vi "FPGA_target_execute_function.vi"(0 "tick_count_in":u32, 2 "data_in":T1, 4 "set_stop_output_in":bool, 5 "input_data_in":u8, 7 "stop_request":bool, 8 "fifo_empty_in":bool, 11 "C1_data":T2) -> (10 "set_output":bool, 12 "read_fifo":bool, 13 "stop":bool, 14 "tick_count_out":u32, 16 "data_dup":T1, 17 "fifo_empty_out":bool, 18 "set_stop_output_out":bool, 19 "input_data_out":u8)   [LabVIEW 2014]
doc: "executes a command (time, wait, jump, stop)"
uses:
  FPGA_32BitPattern_data_type.ctl
  FPGA_cmd_data_type.ctl
  <vilib>/rvi/eio/common/nirviEmuTemplateMethod_errors.vi
  <vilib>/eio/EIONode/EIONode.xnode
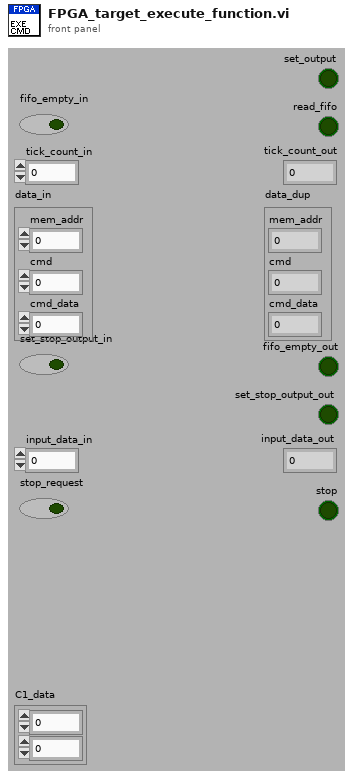
[diagram p1: front panel]
types:
  T1 = typedef "FPGA_cmd_data_type.ctl" = cluster{"mem_addr":u32, "cmd":u8, "cmd_data":u32}
  T2 = typedef "FPGA_32BitPattern_data_type.ctl" = cluster{"port0":u8, "port1":u8}
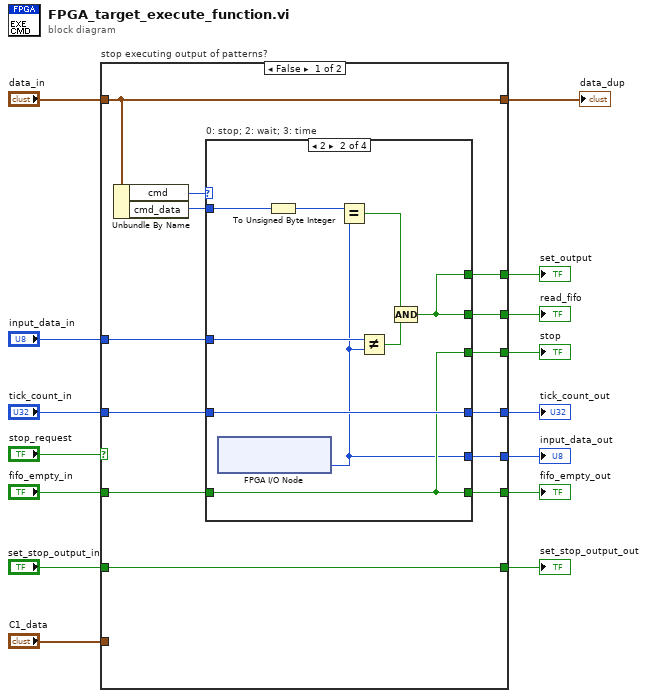
[diagram p0: block diagram]
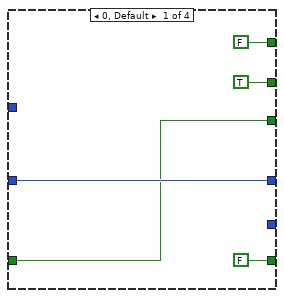
[diagram p2: hidden frame]
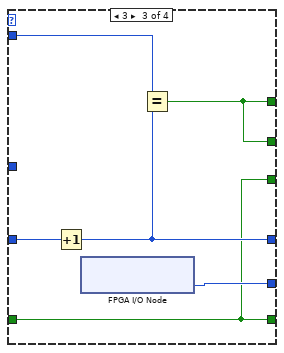
[diagram p3: hidden frame]
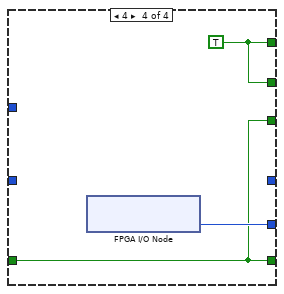
[diagram p4: hidden frame]
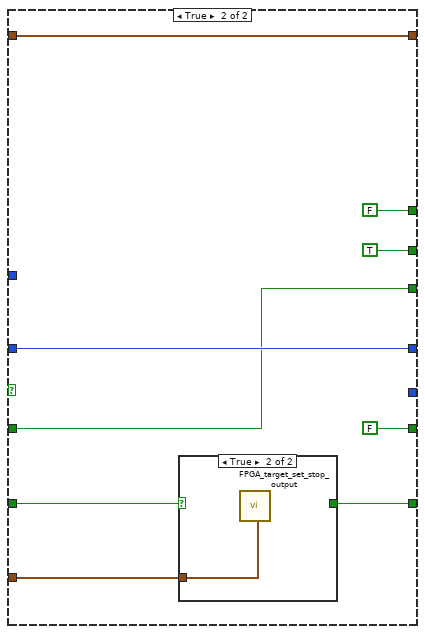
[diagram p5: hidden frame]
diagram:
  n1 = case "stop executing output of patterns?" shown="False" "stop_request" {
    tunnel: "tick_count_in" -> [w28 w59]
    tunnel: [w27 FALSE] -> w14
    tunnel: [w26 w59] -> w13
    tunnel: [w25 w53] -> w12
    tunnel: "fifo_empty_in" -> [w21 w53]
    tunnel: [w16 TRUE] -> w9
    tunnel: [w24 _] -> w8
    tunnel: "input_data_in" -> [w23 _]
    tunnel: "set_stop_output_in" -> [w22 w57]
    tunnel: "C1_data" -> [_ w56]
    tunnel: [w22 w55] -> w4
    tunnel: "data_in" -> [w20 w54]
    tunnel: [w20 w54] -> w2
    tunnel: [w17 FALSE ("fifo_empty_in")] -> w1
    frame False {
      n2 = Unbundle By Name(w20) -> ("cmd"=w19:u8, "cmd_data"=w18:u32)
      n3 = case "0: stop; 2: wait; 3: time" shown="2" w19 {
        tunnel: w18 -> [_ w39 w48 _]
        tunnel: w28 -> [w33 w42 w46 _]
        tunnel: [FALSE w36 w43 w49] -> w27
        tunnel: [w33 w42 w45 _] -> w26
        tunnel: [w31 w37 w44 w50] -> w25
        tunnel: [_ w34 w47 w51] -> w24
        tunnel: w23 -> [_ w35 _ _]
        tunnel: w21 -> [w31 w37 w44 w50]
        tunnel: [FALSE ("fifo_empty_in") w37 w44 w50] -> w17
        tunnel: [TRUE ("fifo_empty") w36 w43 w49] -> w16
        frame 0, Default {
        }
        frame 2 {
          n4 = xnode ("FPGA I/O Node")() -> ("TriggerIn_0-7"=w34:u8)  [unwired: 1 in, 1 out]
          n5 = To Unsigned Byte Integer(number=w39) -> (unsigned 8bit integer=w40:u8)
          n6 = Equal?(x=w40, y=w34) -> (x = y?=w41:bool)
          n7 = Not Equal?(x=w35, y=w34) -> (x != y?=w38:bool)
          n8 = Compound Arithmetic op=AND(w41, w38) -> (w36:bool)
        }
        frame 3 {
          n9 = Increment(x=w46) -> (x+1=w45:u32)
          n10 = xnode ("FPGA I/O Node")() -> ("TriggerIn_0-7"=w47:u8)  [unwired: 1 in, 1 out]
          n11 = Equal?(x=w48, y=w45) -> (x = y?=w43:bool)
        }
        frame 4 {
          w49 = TRUE
          n12 = xnode ("FPGA I/O Node")() -> ("TriggerIn_0-7"=w51:u8)  [unwired: 1 in, 1 out]
        }
      }
    }
    frame True {
      n13 = case shown="True" w57 {
        selector: w57 -> [w61 _]
        tunnel: w56 -> [_ w62]
        tunnel: [w61 _] -> w55
        frame False {
        }
        frame True {
          n14 = call "FPGA_target_set_stop_output.vi"("connector1_data"=w62) -> ()  [unwired: 19 in]
        }
      }
    }
  }
  "set_output" <- w14
  "tick_count_out" <- w13
  "stop" <- w12
  "read_fifo" <- w9
  "input_data_out" <- w8
  "set_stop_output_out" <- w4
  "data_dup" <- w2
  "fifo_empty_out" <- w1
